vi "WhereExit.vi"(7 "Block Array":dbl[][](array[numeric]), 8 "Block Color":dbl[][](array[numeric]), 9 "Proc Block Index":i16) -> (0 "Target Index":i32, 2 "Target POS":dbl[](array[numeric]))   [LabVIEW 2018]
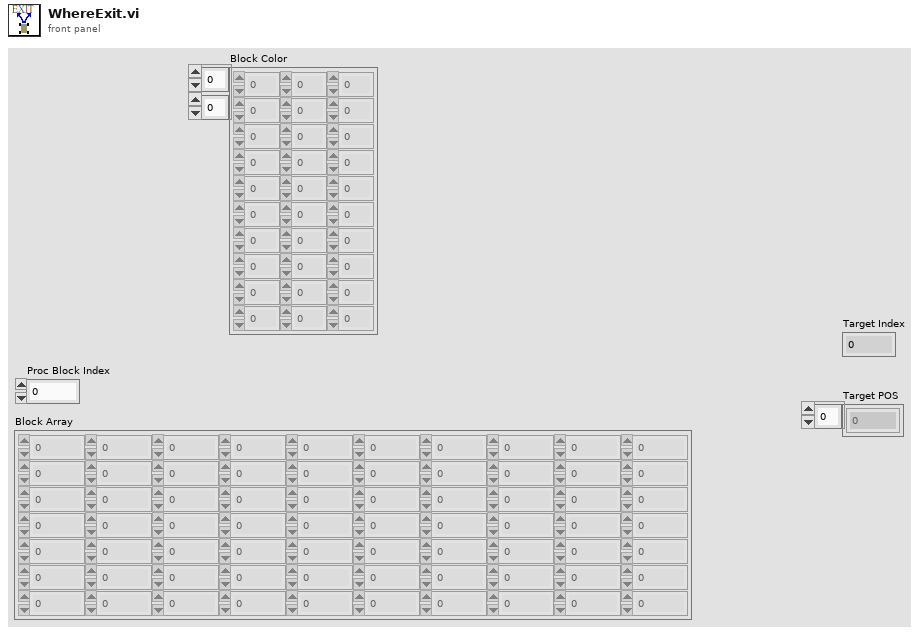
[diagram p1: front panel]
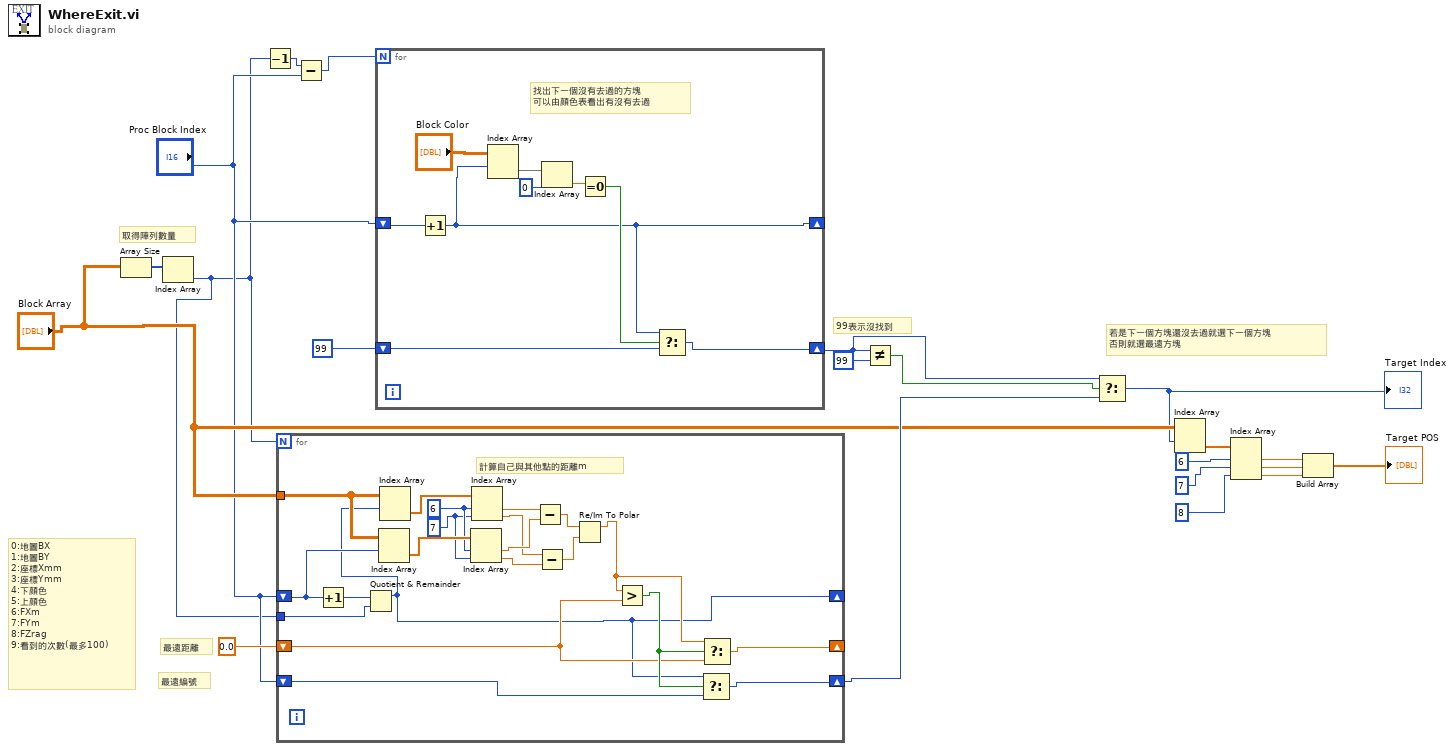
[diagram p0: block diagram]
diagram:
  # "99表示沒找到"
  # "若是下一個方塊還沒去過就選下一個方塊\n否則就選最遠方塊"
  # "最遠編號"
  # "最遠距離"
  # "取得陣列數量"
  # "0:地圖BX\n1:地圖BY\n2:座標Xmm\n3:座標Ymm\n4:下顏色\n5:上顏色\n6:FXm\n7:FYm\n8:FZrag\n9:看到的次數(最多100)"
  n1 = Array Size(array="Block Array") -> (size(s)=w21:i32[])
  n2 = Index Array(array=w21) -> (element=w2:i32)  [unwired: 1 in]
  n3 = Decrement(x=w2) -> (x-1=w1:i32)
  n4 = for {
    N: w2 -> [_]
    shift-right: [w22] -> _
    shift-left: "Proc Block Index" -> [w39]
    shift-right: [w26] -> _
    shift-left: 0.0 -> [w27]
    tunnel: "Block Array" -> [w40]
    tunnel: w2 -> [w42]
    shift-right: [w23] -> w19
    shift-left: "Proc Block Index" -> [w24]
    w36 = 7 ("index")
    w37 = 6 ("index")
    # "計算自己與其他點的距離m"
    n5 = Increment(x=w39) -> (x+1=w25:i32)
    n6 = Quotient & Remainder(x=w25, y=w42) -> (x-y*floor(x/y)=w22:i32)  [unwired: 1 out]
    n7 = Index Array(array=w40, index (row)=w39) -> (element=w38:dbl[])  [unwired: 1 in]
    n8 = Index Array(array=w40, index (row)=w22) -> (element=w41:dbl[])  [unwired: 1 in]
    n9 = Index Array(array=w38, index #1=w37, index #2=w36) -> (element #1=w34:dbl, element #2=w32:dbl)
    n10 = Index Array(array=w41, index #1=w37, index #2=w36) -> (element #1=w35:dbl, element #2=w33:dbl)
    n11 = Subtract(x=w35, y=w34) -> (x-y=w31:dbl)
    n12 = Subtract(x=w33, y=w32) -> (x-y=w30:dbl)
    n13 = Re/Im To Polar(2:w30, 3:w31) -> (1:w28:dbl)  [unwired: 1 out]
    n14 = Greater?(x=w28, y=w27) -> (0:w29:bool)
    n15 = Select(t=w22, s=w29, f=w24) -> (s? t:f=w23:i32)
    n16 = Select(t=w28, s=w29, f=w27) -> (s? t:f=w26:dbl)
  }
  n17 = Subtract(x=w1, y="Proc Block Index") -> (x-y=w7:i32)
  n18 = for {
    N: w7 -> [_]
    shift-right: [w44] -> _
    shift-left: "Proc Block Index" -> [w51]
    shift-right: [w43] -> w3
    shift-left: 99 -> [w45]
    # "找出下一個沒有去過的方塊\n可以由顏色表看出有沒有去過"
    n19 = Increment(x=w51) -> (x+1=w44:i16)
    n20 = Index Array(array="Block Color", index (row)=w44) -> (element=w49:dbl[])  [unwired: 1 in]
    n21 = Index Array(array=w49, index=0) -> (element=w47:dbl)
    n22 = Equal To 0?(x=w47) -> (x = 0?=w46:bool)
    n23 = Select(t=w44, s=w46, f=w45) -> (s? t:f=w43:i32)
  }
  n24 = Not Equal?(x=w3, y=99) -> (x != y?=w4:bool)
  n25 = Select(t=w3, s=w4, f=w19) -> (s? t:f=w17:i32)
  "Target Index" <- w17
  n26 = Index Array(array="Block Array", index (row)=w17) -> (element=w16:dbl[])  [unwired: 1 in]
  n27 = Index Array(array=w16, index #1=6 ("index"), index #2=7 ("index"), index #3=8 ("index")) -> (element #1=w12:dbl, element #2=w11:dbl, element #3=w10:dbl)
  n28 = Build Array(w12, w11, w10) -> (→"Target POS":dbl[])
